vi "uc480_ArrayToImage_v4.vi"(8 "Error In":errorcluster, 10 "InArray":u8[](array[numeric]), 11 ".NET (Reference)":refnum<k24>) -> (0 "Error Out":errorcluster, 2 "Image":picture, 3 ".NET (Reference) 2":refnum<k24>)   [LabVIEW 2018]
doc: "ArrayToVision converts 24/32-bit one-dimensional arrays to a two-dimensional U32 array."
uses:
  C:/Program Files/National Instruments/LabVIEW 2018/uc480DotNet.dll
  uc480DotNet.dll
  <vilib>/picture/picture.llb/Draw True-Color Pixmap.vi
panel:
  # "Input"
  # "Output"
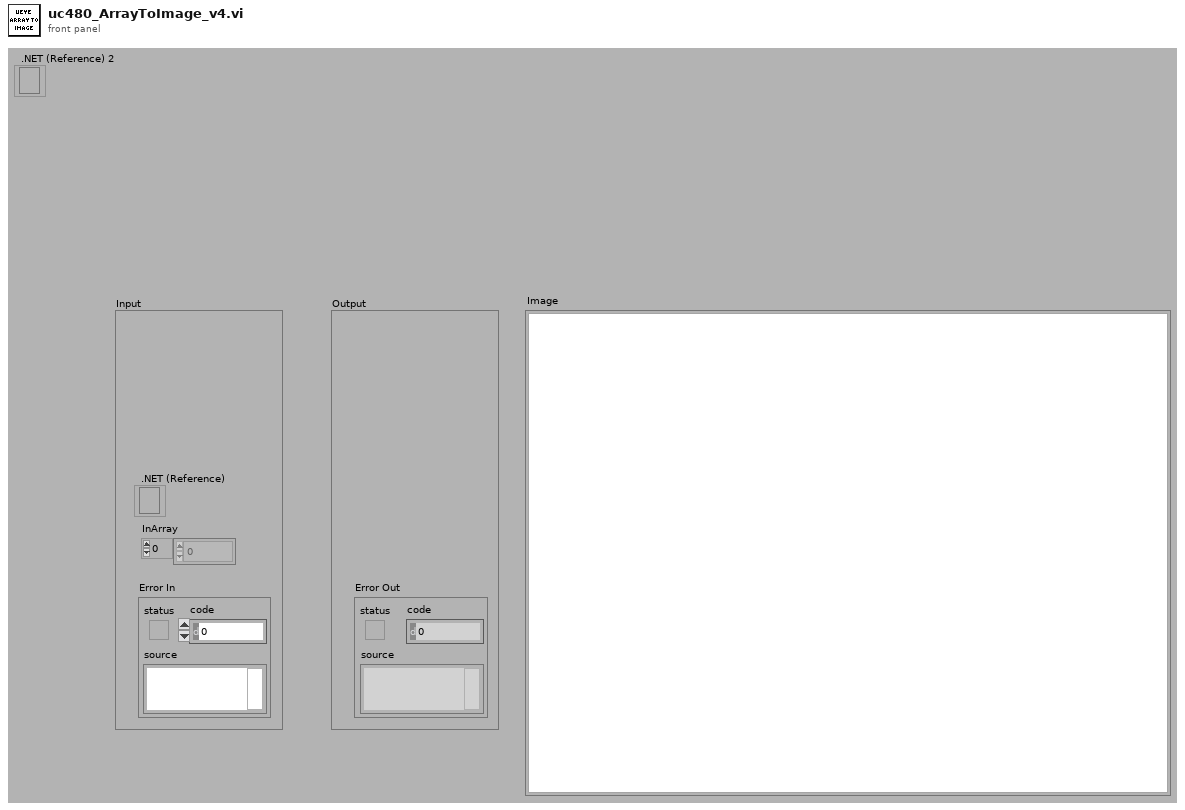
[diagram p1: front panel]
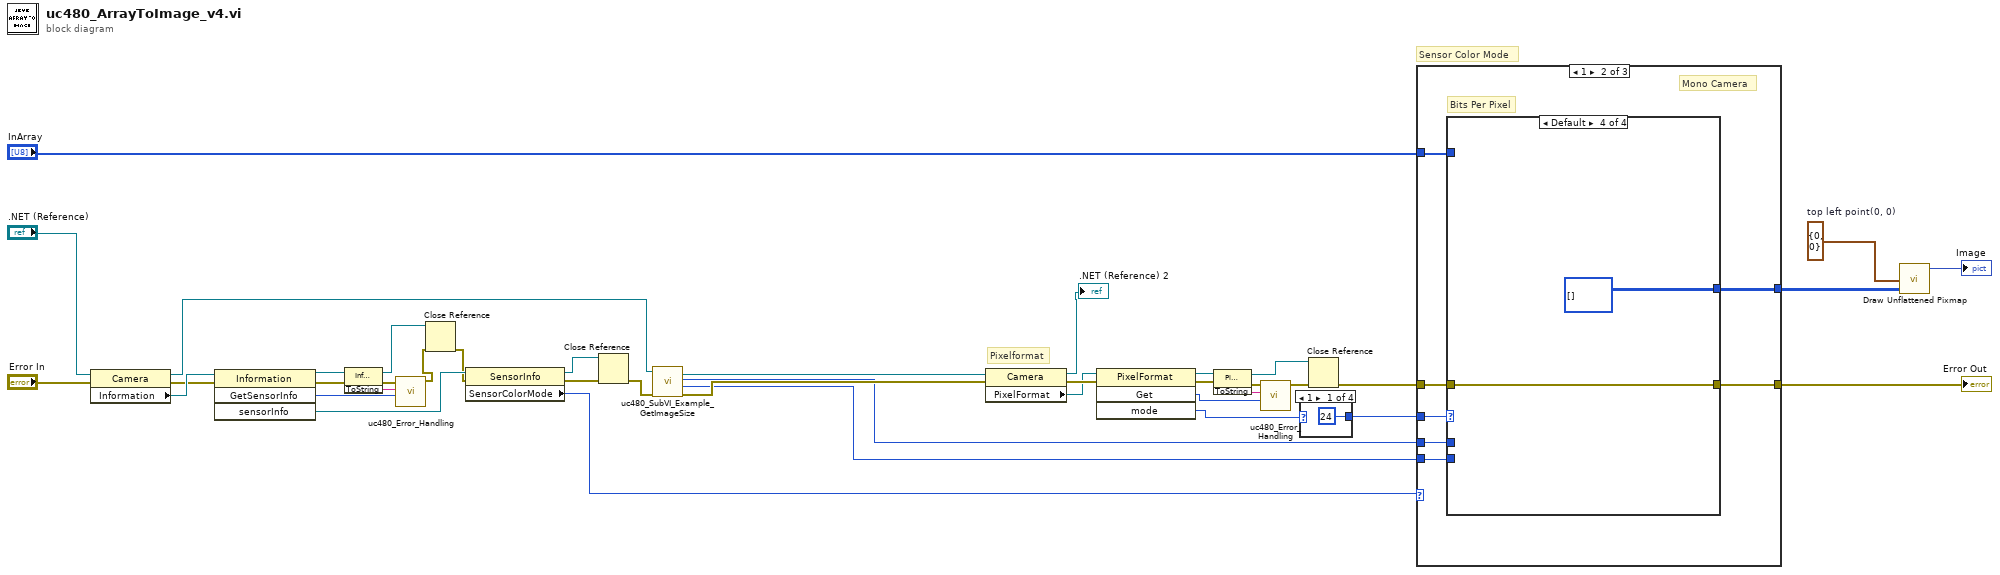
[diagram p0: block diagram]
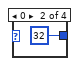
[diagram p2: hidden frame]
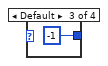
[diagram p3: hidden frame]
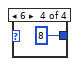
[diagram p4: hidden frame]
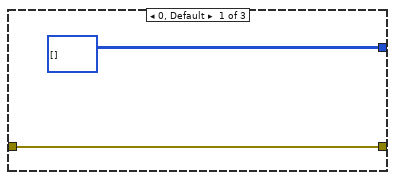
[diagram p5: hidden frame]
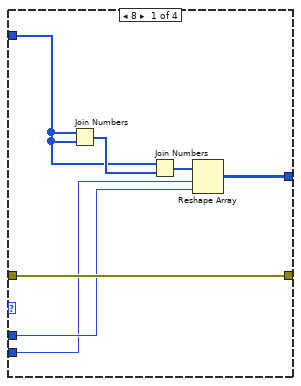
[diagram p6: hidden frame]
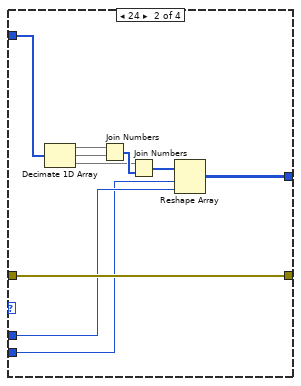
[diagram p7: hidden frame]
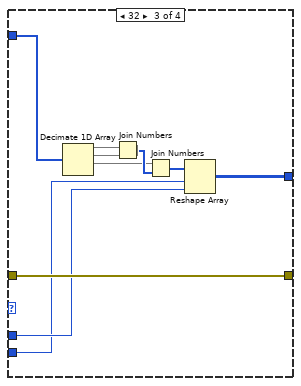
[diagram p8: hidden frame]
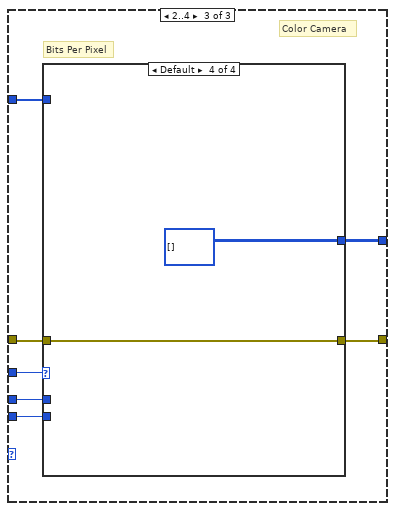
[diagram p9: hidden frame]
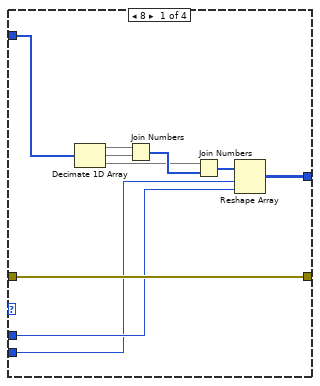
[diagram p10: hidden frame]
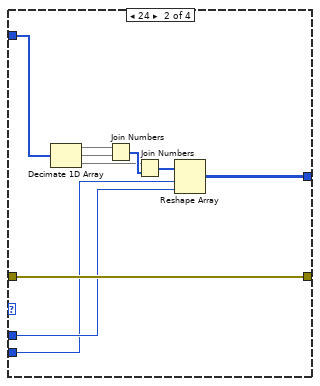
[diagram p11: hidden frame]
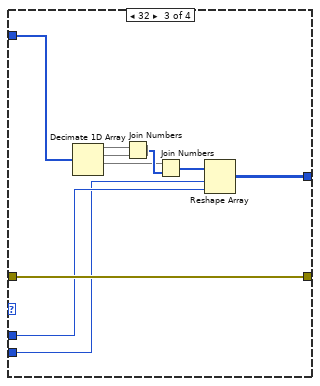
[diagram p12: hidden frame]
diagram:
  w40 = cluster{i16, i16} {0, 0}  # top left point(0, 0)
  # "Sensor Color Mode"
  # "Pixelformat"
  n1 = property on="Eigenschaftsknoten" class="Camera"(reference=".NET (Reference)", error in="Error In") -> (reference out=w2:refnum<k24>, error out=w35:errorcluster, "Information"=w38:refnum<k24>)
  n2 = invoke class="Information" method="GetSensorInfo"(reference=w38, error in=w35) -> (reference out=w30:refnum<k24>, error out=w29:errorcluster, "GetSensorInfo"=w28:i32, "sensorInfo"=w37:refnum<k24>)  [unwired: 2 in]
  n3 = invoke class="Information" method="ToString"(reference=w30, error in=w29) -> (reference out=w11:refnum<k24>, error out=w32:errorcluster, "ToString"=w31:string)  [unwired: 1 in]
  n4 = call <instrlib>:"uc480_Error_Handling.vi"("Error Code"=w28, "Error String"=w31, "Error In"=w32) -> ("Error Out"=w10:errorcluster)  [unwired: 8 in]
  n5 = Close Reference(reference=w11, error in (no error)=w10) -> (error out=w9:errorcluster)
  n6 = property class="SensorInfo"(reference=w37, error in=w9) -> (reference out=w8:refnum<k24>, error out=w7:errorcluster, "SensorColorMode"=w36:i32)
  n7 = Close Reference(reference=w8, error in (no error)=w7) -> (error out=w6:errorcluster)
  n8 = call <instrlib>:"uc480_SubVI_Example_GetImageSize.vi"("Error In"=w6, ".NET (Reference)"=w2) -> ("Error Out"=w16:errorcluster, "Height"=w12:i32, "Width"=w13:i32, ".NET (Reference)"=w14:refnum<k24>)  [unwired: 6 in]
  n9 = property class="Camera"(reference=w14, error in=w16) -> (reference out=→".NET (Reference) 2":refnum<k24>, error out=w22:errorcluster, "PixelFormat"=w21:refnum<k24>)
  n10 = invoke class="PixelFormat" method="Get"(reference=w21, error in=w22) -> (reference out=w27:refnum<k24>, error out=w26:errorcluster, "Get"=w25:i32, "mode"=w20:i32)  [unwired: 2 in]
  n11 = invoke class="PixelFormat" method="ToString"(reference=w27, error in=w26) -> (reference out=w5:refnum<k24>, error out=w23:errorcluster, "ToString"=w24:string)  [unwired: 1 in]
  n12 = call <instrlib>:"uc480_Error_Handling.vi"("Error Code"=w25, "Error String"=w24, "Error In"=w23) -> ("Error Out"=w4:errorcluster)  [unwired: 8 in]
  n13 = case shown="1" w20 {
    tunnel: [24 32 -1 8] -> w19
    frame 1 {
    }
    frame 0 {
    }
    frame Default {
    }
    frame 6 {
    }
  }
  n14 = Close Reference(reference=w5, error in (no error)=w4) -> (error out=w3:errorcluster)
  n15 = case shown="1" w36 {
    tunnel: "InArray" -> [_ w50 w89]
    tunnel: w13 -> [_ w48 w84]
    tunnel: w12 -> [_ w47 w83]
    tunnel: w19 -> [_ w49 w85]
    tunnel: w3 -> [w45 w53 w86]
    tunnel: [w45 w52 w87] -> w18
    tunnel: [u32[][] [] w51 w88] -> w17
    frame 0, Default {
    }
    frame 1 {
      # "Bits Per Pixel"
      # "Mono Camera"
      n16 = case shown="Default" w49 {
        tunnel: w50 -> [w56 w65 w74 _]
        tunnel: w47 -> [w54 w61 w71 _]
        tunnel: w48 -> [w55 w62 w72 _]
        tunnel: [w60 w64 w75 u32[][] []] -> w51
        tunnel: w53 -> [w59 w63 w73 w81]
        tunnel: [w59 w63 w73 w81] -> w52
        frame 8 {
          n17 = Join Numbers(hi=w56, lo=w56) -> ((hi.lo)=w58:u16[])
          n18 = Join Numbers(hi=w56, lo=w58) -> ((hi.lo)=w57:u32[])
          n19 = Reshape Array(w57, w54, w55) -> (w60:u32[][])
        }
        frame 24 {
          n20 = Decimate 1D Array(w65) -> (w70:u8[], w69:u8[], w67:u8[])
          n21 = Join Numbers(hi=w69, lo=w70) -> ((hi.lo)=w68:u16[])
          n22 = Join Numbers(hi=w67, lo=w68) -> ((hi.lo)=w66:u32[])
          n23 = Reshape Array(w66, w61, w62) -> (w64:u32[][])
        }
        frame 32 {
          n24 = Decimate 1D Array(w74) -> (w80:u8[], w79:u8[], w77:u8[])  [unwired: 1 out]
          n25 = Join Numbers(hi=w79, lo=w80) -> ((hi.lo)=w78:u16[])
          n26 = Join Numbers(hi=w77, lo=w78) -> ((hi.lo)=w76:u32[])
          n27 = Reshape Array(w76, w71, w72) -> (w75:u32[][])
        }
        frame Default {
        }
      }
    }
    frame 2..4 {
      # "Bits Per Pixel"
      # "Color Camera"
      n28 = case shown="Default" w85 {
        tunnel: w89 -> [w91 w104 w113 _]
        tunnel: w83 -> [w96 w100 w110 _]
        tunnel: w84 -> [w97 w101 w111 _]
        tunnel: [w99 w103 w114 u32[][] []] -> w88
        tunnel: w86 -> [w98 w102 w112 w120]
        tunnel: [w98 w102 w112 w120] -> w87
        frame 8 {
          n29 = Decimate 1D Array(w91) -> (w95:u8[], w94:u8[], w92:u8[])
          n30 = Join Numbers(hi=w94, lo=w95) -> ((hi.lo)=w93:u16[])
          n31 = Join Numbers(hi=w92, lo=w93) -> ((hi.lo)=w90:u32[])
          n32 = Reshape Array(w90, w96, w97) -> (w99:u32[][])
        }
        frame 24 {
          n33 = Decimate 1D Array(w104) -> (w109:u8[], w108:u8[], w106:u8[])
          n34 = Join Numbers(hi=w108, lo=w109) -> ((hi.lo)=w107:u16[])
          n35 = Join Numbers(hi=w106, lo=w107) -> ((hi.lo)=w105:u32[])
          n36 = Reshape Array(w105, w100, w101) -> (w103:u32[][])
        }
        frame 32 {
          n37 = Decimate 1D Array(w113) -> (w119:u8[], w118:u8[], w116:u8[])  [unwired: 1 out]
          n38 = Join Numbers(hi=w118, lo=w119) -> ((hi.lo)=w117:u16[])
          n39 = Join Numbers(hi=w116, lo=w117) -> ((hi.lo)=w115:u32[])
          n40 = Reshape Array(w115, w110, w111) -> (w114:u32[][])
        }
        frame Default {
        }
      }
    }
  }
  "Error Out" <- w18
  n41 = call-poly <vilib>:"Draw Unflattened Pixmap.vi"("top left point(0, 0)"=w40, "data (RGB format)"=w17) -> ("new picture"=→"Image":picture)  [unwired: 7 in]
